vi "DefaultSamples.vi"(3 "Defaults":cluster{"name":string, "Content":string}[](array[cluster]), 6 "error in (no error)":errorcluster, 9 "Task":enum16{"Load to VI", "Save to Disk"}(ring), 11 "path (use dialog)":path=path "/Users/crogers/Dropbox (Rogers)/Documents/Violin/ViolinData/Samples") -> (1 "No Errors?":bool)   [LabVIEW 2022 SP3]
panel:
  out "Array":T1(array[cluster])
  # "You should run this to grab all the files from the\nDetault Settings and put them in the array below so that\nwhen people run and do not have a Violin Compare folder\nthey will get it pre-poulated with these."
  # "defaults is hidden - much faster VI update reates."
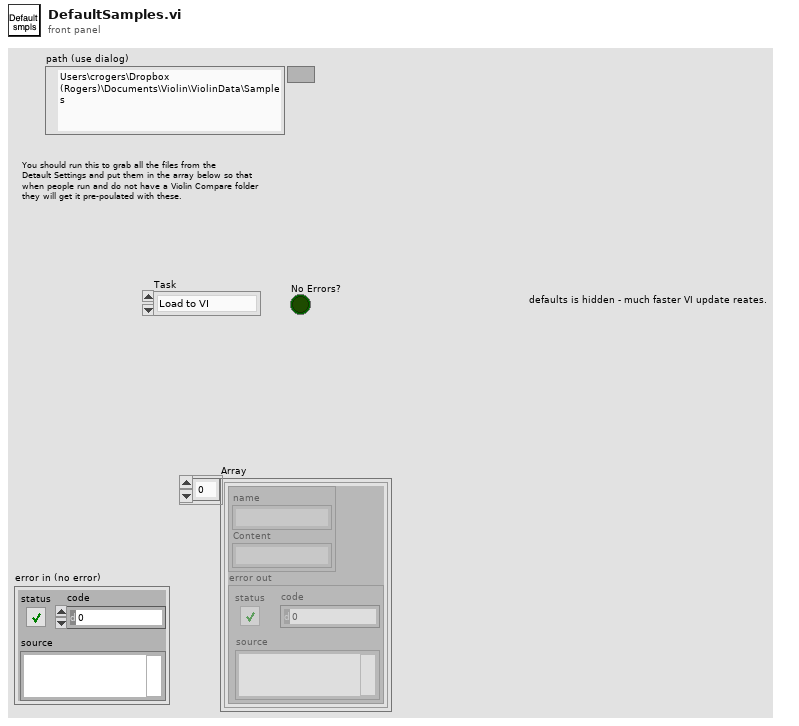
[diagram p1: front panel]
types:
  T1 = cluster{cluster{"name":string, "Content":string}, "error out":errorcluster}[]
  T2 = cluster{cluster{"name":string, "Content":string}, "error out":errorcluster}
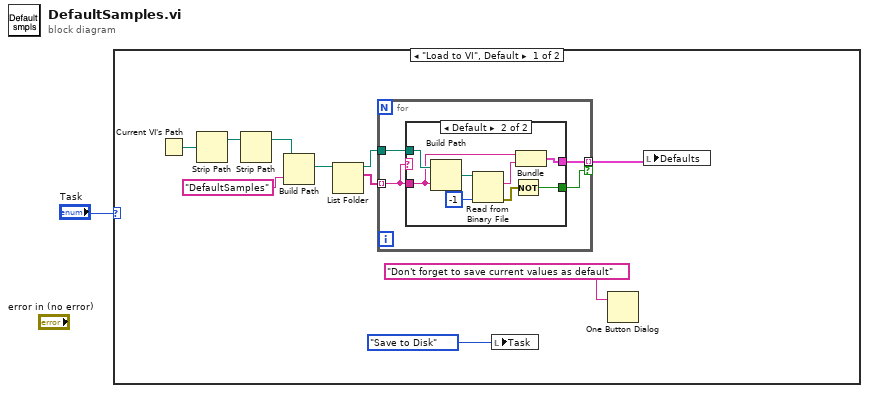
[diagram p0: block diagram]
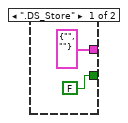
[diagram p2: hidden frame]
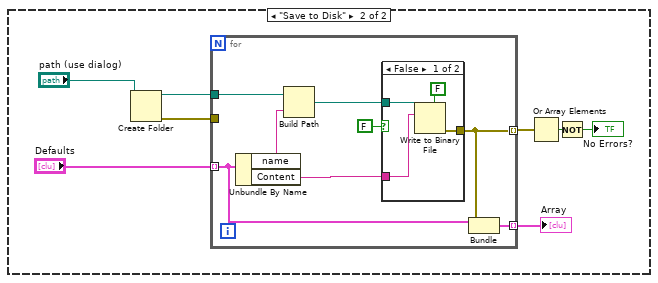
[diagram p3: hidden frame]
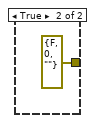
[diagram p4: hidden frame]
diagram:
  n1 = case shown="\"Load to VI\", Default" "Task" {
    frame "Load to VI", Default {
      n2 = Current VI's Path() -> (path=w11:path)
      n3 = Strip Path(path=w11) -> (stripped path=w10:path)  [unwired: 1 out]
      n4 = Strip Path(path=w10) -> (stripped path=w8:path)  [unwired: 1 out]
      n5 = Build Path(base path=w8, name or relative path="DefaultSamples") -> (appended path=w5:path)
      n6 = List Folder(path=w5) -> (path out=w6:path, filenames=w7:string[])  [unwired: 3 in, 2 out]
      n7 = for {
        tunnel: w7 -> [w12] mode=indexing
        tunnel: w6 -> [w15]
        tunnel: [w14] -> w4 mode=indexing if=w13
        n8 = case shown="Default" w12 {
          tunnel: w15 -> [_ w25]
          tunnel: w12 -> [_ w22]
          tunnel: [cluster{string, string} {"", ""} w21] -> w14
          tunnel: [FALSE w19] -> w13
          frame ".DS_Store" {
          }
          frame Default {
            n9 = Build Path(base path=w25, name or relative path=w22) -> (appended path=w24:path)
            n10 = Read from Binary File(10:-1 ("count (1)"), 11:w24) -> (0:w20:errorcluster, 2:w23:string)  [unwired: 4 in, 2 out]
            n11 = Not(x=w20) -> (.not. x?=w19:bool)
            n12 = Bundle(w22, w23) -> (w21:cluster{string, string})  [unwired: 1 in]
          }
        }
      }
      n13 = local write "Task"(enum16{"Load to VI", "Save to Disk"}."Save to Disk" ("Task")) -> ()
      n14 = One Button Dialog(message="Don't forget to save current values as default") -> ()  [unwired: 1 in, 1 out]
      n15 = local write "Defaults"(w4) -> ()
    }
    frame "Save to Disk" {
      n16 = Create Folder(path (use dialog)="path (use dialog)") -> (created path=w32:path, error out=w30:errorcluster)  [unwired: 2 in, 1 out]
      n17 = for {
        tunnel: w32 -> [w41]
        tunnel: "Defaults" -> [w36] mode=indexing
        tunnel: [w35] -> w29 mode=indexing
        tunnel: w30 -> [_]
        tunnel: [w34] -> w27 mode=indexing
        n18 = Unbundle By Name(w36) -> ("name"=w40:string, "Content"=w39:string)
        n19 = Build Path(base path=w41, name or relative path=w40) -> (appended path=w38:path)
        n20 = case shown="False" FALSE {
          tunnel: w39 -> [w45 _]
          tunnel: [w44 errorcluster {"status"=FALSE, "code"=0, "source"=""} ("error out")] -> w35
          tunnel: w38 -> [w43 _]
          frame False {
            n21 = Write to Binary File(file (use dialog)=w43, data=w45, 5:FALSE ("prepend array or string size? (T)")) -> (error out=w44:errorcluster)  [unwired: 3 in, 2 out]
          }
          frame True {
          }
        }
        n22 = Bundle(w36, "error out"=w35) -> (w34:T2)  [unwired: 1 in]
      }
      "Array" <- w27
      n23 = Or Array Elements(Boolean array=w29) -> (logical OR=w28:bool)
      n24 = Not(x=w28) -> (.not. x?=→"No Errors?":bool)
    }
  }
